vi "pH meter copyright.vi"   [LabVIEW 2010]
panel:
  # "pH meter\nbased on Data Server Technology"
  # "©2004 Monroe Weber-Shirk\nall rights reserved\nmw24@cornell.edu\n\n\nCivil and Environmental Engineering\nCornell University"
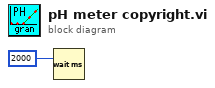
[diagram p0: block diagram]
diagram:
  n1 = Wait (ms)(milliseconds to wait=2000) -> ()  [unwired: 1 out]
